vi "histo_maint.vi"(8 "Error in (no error)":errorcluster, 11 "Connection In":refnum<k7>) -> (0 "Error out":errorcluster, 2 "Table":string[][](table), 3 "Connection Out":refnum<k7>)   [LabVIEW 2019]
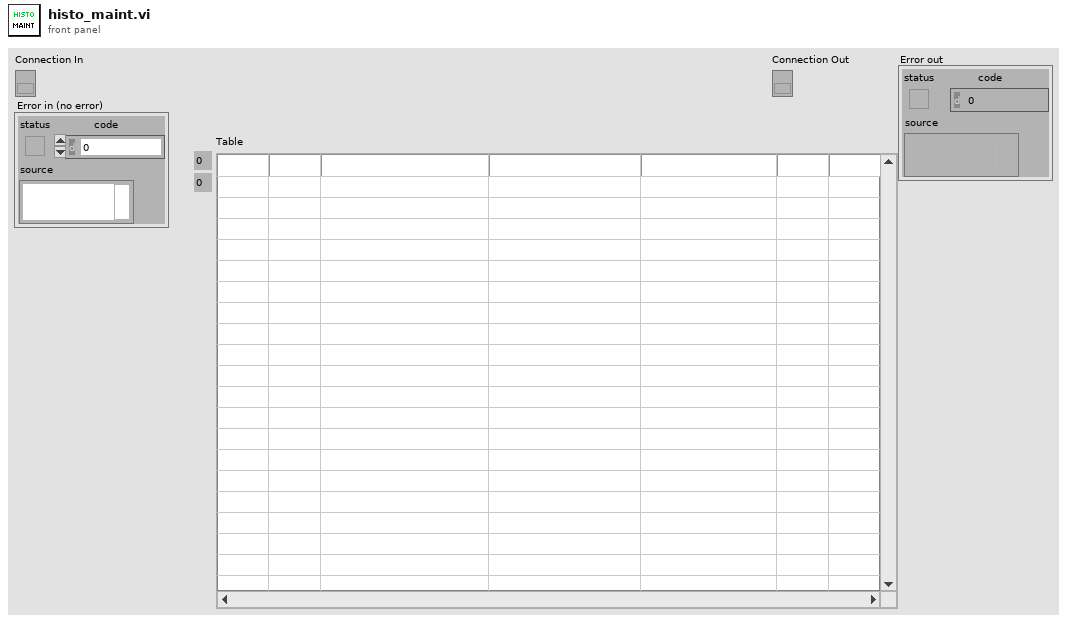
[diagram p1: front panel]
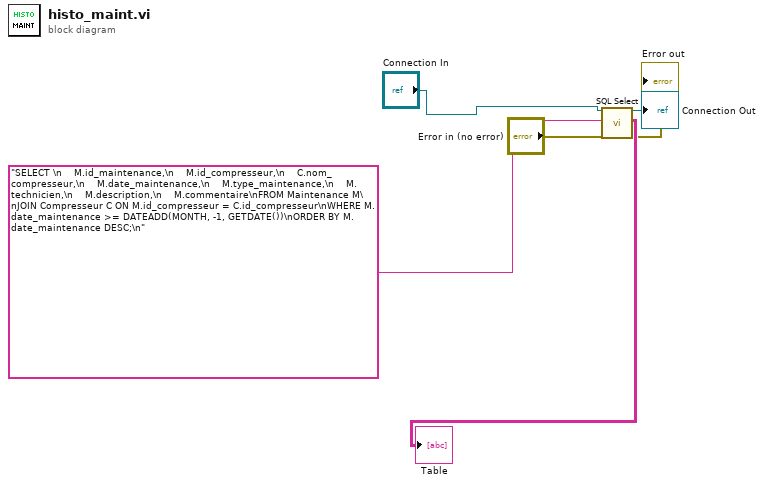
[diagram p0: block diagram]
diagram:
  n1 = call <vilib>:"SQL Select.vi"("Connection In"="Connection In", "SQL Query"="SELECT \n    M.id_maintenance,\n    M.id_compresseur,\n    C.nom_compresseur,\n    M.date_maintenance,\n    M.type_maintenance,\n    M.technicien,\n    M.description,\n    M.commentaire\nFROM Maintenance M\nJOIN Compresseur C ON M.id_compresseur = C.id_compresseur\nWHERE M.date_maintenance >= DATEADD(MONTH, -1, GETDATE())\nORDER BY M.date_maintenance DESC;\n", "Error in (no error)"="Error in (no error)") -> ("Connection Out"=→"Connection Out":refnum<k7>, "Data"=→"Table":string[][], "Error out"=→"Error out":errorcluster)  [unwired: 14 in]
